vi "Main_13a.vi"() -> ()   [LabVIEW 2023]
panel:
  out "Array":cluster{"Array":bool[][]}[](array[cluster])
  out "Answer":i32
  in  "Puzzle":string=".####.#...##.#.\n...###.##.#.#..\n...###.##.#.#..\n.####.#...#..#.\n..##......#..#.\n#.#...#.##...##\n.#.#.#..##..##.\n#..##...#####.#\n.#.#.#.#..##.#.\n.....###.#.#..#\n.....###.#.#..#\n\n.#.###.....\n#..#.##...#\n.#.....#.#.\n.#.....#.#.\n#..#.##...#\n.#.###.....\n##.#..##.##\n#....##..#.\n.##.##.#.##\n...#..###.#\n...#..###.#\n.##.##.#.##\n#....##..#.\n####..##.##\n.#.###.....\n#..#.##...#\n.#.....#.#.\n\n###....##....\n####..#..#..#\n..###.####.##\n..#..######..\n...#.######.#\n#####.#.##.##\n##.#..#..#..#\n##....####...\n....#......#.\n.....#.##.#..\n##...##..##..\n...##.#..#.##\n##..###..###.\n\n.##.#...##.\n.#.########\n.##.#.#.##.\n#.##..#....\n####.##....\n####.##....\n#.##..#....\n.##.#.#.##.\n.#.########\n.##.#...##.\n..####.####\n.##.###.###\n.#..#.#.##.\n#.####..##.\n...#..#....\n\n.....##..#.\n.##..##.#.#\n#..#...####\n####.....##\n#..#.##....\n#####.....#\n#####.....#\n#..#.##....\n####.#...##\n#..#...####\n.##..##.#.#\n.....##..#.\n....##.##..\n\n#####..\n.##.#..\n.##....\n.##...#\n.##....\n#..####\n..#.#.#\n#####..\n#####.#\n.##...#\n.##.##.\n.##.##.\n.##...#\n\n.##.#.##.##.##.##\n.##.####....###..\n.##.#.#.#.##..##.\n#..#.#..#.#.##.#.\n....####...####..\n#..##.#...######.\n....#.#..........\n#..#.##.####..###\n#####...##......#\n....###..##.##.##\n####..###..####..\n.##..##..#.####.#\n#..##..##..#..#..\n.##..#.#.#..##..#\n####..####.####.#\n####.....###..###\n#..#..##.##.##.##\n\n.#..#.#.#####\n#.##.#.#.#.##\n#.##.#.#.#.##\n.#..#.#.#.###\n##..##..###..\n##.####.#####\n.##.#.#...###\n\n.###.#.###.###..#\n...####.####..#.#\n#..####.####..#.#\n.###.#.###.###..#\n...###..#..##....\n.#.#####.###..###\n#.#.#####.#.#####\n.##.###.#...###..\n.##.#.....##..##.\n#..##.####...##..\n#.#.#..#....#.###\n..#...#...##..##.\n##..#.######...##\n###.#.####..#..##\n...#..##..##...##\n###....##.#..#..#\n###....##.#..#..#\n\n##.###..####..#\n#.###.###.##..#\n..##...##..##.#\n..##...##..##.#\n#.###.###.##..#\n##.###..####..#\n....#####.#####\n##..#....#.#..#\n##.#..#.#...#..\n.##.#..##.#.###\n.##.#..##.#.###\n#..#..#.#...#..\n##..#....#.#..#\n\n.###.#....##....#\n#.##.##........##\n...###.#..##..#.#\n...###.#..##..#.#\n#.##.##........##\n.###.#....##....#\n.###..#.##..##.#.\n.###.#...####...#\n####.....####....\n###...##...#..##.\n.#..#.#.#.##.#.#.\n\n#.#..#.\n#.#..#.\n#......\n###..##\n##.##.#\n..####.\n#......\n##.....\n.##..##\n..#..#.\n..#..#.\n.##..##\n...##..\n\n##.#########..##.\n...#.####.#.##..#\n##.#...#..##..##.\n....#..###.##.#.#\n....#..###.##.#.#\n##.#...#..#...##.\n...#.####.#.##..#\n##.#########..##.\n##...####...##...\n###...##..###.#.#\n...#.#..##.#.....\n.........#####...\n....##..#.#.##.##\n...#.#.###.....#.\n...##..#.##.#.#.#\n##...##....#.####\n###....###......#\n\n..##.##.##......#\n.###....###....##\n#.###..###.####.#\n.##########.##.##\n...##..##........\n###......###..###\n.##########....##\n.#.######.#.##.#.\n.....##.....##...\n####.##.####..###\n...#....#........\n.##.#..#.##.....#\n..##.##.##......#\n\n####.##\n.##..#.\n..###.#\n.##.#.#\n###.#..\n##...##\n##...##\n#####..\n.##.#.#\n..###.#\n.##..#.\n####.##\n####.##\n.##..#.\n..###.#\n\n#.###..\n.....##\n..#....\n.#.##..\n..#.###\n..#..##\n.#.##..\n\n#..#.###....#####\n##.####.####.####\n#...###..#..#.##.\n..###.#.##.....#.\n..#....####..####\n...#.###.#.##.##.\n.#...###.#..#####\n.#.#...##.#......\n.##.##..#.....##.\n.#..#.#...##.#..#\n.#....##.##.##..#\n###..####.###....\n###..####.###....\n\n######.#.##....\n.####.#..##.##.\n.####.##..#....\n.####.#.#.#####\n#....#..####..#\n.####...#.#....\n..........##..#\n..##..#.#####.#\n######.#...####\n#.##.##.....##.\n.#..#...##.####\n..........#####\n#.##.#####.#..#\n\n#####.#\n##.##.#\n#.#.###\n...##.#\n######.\n......#\n......#\n######.\n...##.#\n#.#.###\n##.##.#\n\n.#..#.#####...#..\n#######.#.#.....#\n#....#...#.#...##\n######...###...##\n.#..#..###..#..##\n#....##..#...##.#\n.####..##.###.##.\n.#..#.##.###..#..\n#....#.#.##.##.#.\n.#..#.#...#.##...\n.####.##.#.#....#\n.......#.##.#.##.\n.......#.##.#.#..\n.####.##.#.#....#\n.#..#.#...#.##...\n\n##.####\n..#....\n###....\n.##....\n#.#....\n#.#....\n..#....\n###.##.\n#..####\n#.#####\n###....\n#..####\n.######\n##.####\n.#.....\n\n###.##....##.##\n##.##......##.#\n####...##...###\n....#.#..#.#...\n....#.....##...\n#####..##..####\n###..##..##..##\n###..#.##.#..##\n###..#....#..##\n#####.####.####\n..#.#..##..#.#.\n..#..#.##.#..#.\n##............#\n\n###.#.##.#.#.#.\n###.#.##.###.#.\n##..#...##....#\n.#..###.###..##\n#.#......###.##\n........##.##.#\n........##.##.#\n#.#......###.##\n.#..###.###..##\n##..#...##....#\n###.#.##.###.#.\n###.#.##.#.#.#.\n.#..#.#...#.###\n.....##.#.##.#.\n.#.###.#.###.##\n.#.#.....###.#.\n##....####.#.##\n\n###......###.\n##.######.###\n###.####.###.\n##..#..#..##.\n..##....##...\n###..##..###.\n####....#####\n####.##.####.\n##.##..##.##.\n#...####...#.\n...#....#....\n...#....#....\n..#.#..#.#..#\n\n.##..##.###..##\n.##.#...##.#.#.\n.##.#...##.#.#.\n.##..##.###..##\n#...#.#..####..\n.#.#....#.#....\n#..##..#..##...\n##....####..#..\n.#.....#.###..#\n..#....#.#...#.\n.##...#.#..#.##\n...##.#..######\n.###.......####\n.###.......####\n...##.#...#####\n\n.#........#.##.\n#.##.#...##.#.#\n###.####...##.#\n###.####..###.#\n#.##.#...##.#.#\n.#........#.##.\n...#.##.#.#.##.\n#.####.###.####\n.#...##.##.###.\n.....#..#.####.\n##.##.##..##..#\n.....#..#.....#\n##.##.#.#####..\n##.##.#.#####..\n.....#..#.....#\n##.##.##..##..#\n.....#..#.####.\n\n######.##.###\n.#..##.##.##.\n#.#.##.##.##.\n#.#..#.##.#..\n....#.####.#.\n#...#..##..#.\n####.#....#.#\n.###.######.#\n####.###.##.#\n....###..###.\n..###.####.##\n..###.####.##\n....###..###.\n\n..##..##..#\n..###.#....\n##....#....\n###.#.#.##.\n##.####.##.\n##...##.##.\n...##..####\n##.#####...\n...#.##....\n..#####.##.\n...#..##..#\n..#.#..####\n##.....####\n...##.#.##.\n..#####.##.\n.....#.#..#\n##.##...##.\n\n#......##.##.##\n..####..#####..\n..#..#...#..#..\n.######.##.#...\n..#..#....#####\n...##....######\n.........#.##..\n.##..##.#......\n####.####.#.###\n\n#......##......##\n..####....####...\n..#..#....#..#..#\n...##......##....\n################.\n.#....#..#....#..\n...##......##....\n.#....#..#....#..\n##....####....##.\n..#..#....#..#...\n..#..#....#..#..#\n##.##.####.##.##.\n###..######..###.\n..####....####...\n...##......##....\n####.######.#####\n.#.##.#..#.##.#.#\n\n...##.##.##..\n##..........#\n##..##..##..#\n..#.######.#.\n##...####...#\n...##.##.##..\n###..####..##\n##...####...#\n...##.#..##..\n....##..##...\n##..#.##.#..#\n\n.#.##.####.##.#..\n##..###..###..##.\n##..##....##..##.\n#.#.##....##.#.#.\n#.#.###..###.#.#.\n##...##..##...###\n#..#.##..##.#..##\n....#.#..#.#....#\n....#.#..#.#.....\n\n.##.#.....#...###\n###..#.####..####\n##....#..####....\n#..###..#.#..####\n..#.####.####.##.\n.##....##...#.##.\n.##....##...#.##.\n..#.####.####.##.\n#..###..#.#..####\n##....#..####....\n###..#.####..####\n\n##..#.#..#.#.\n##.###.##.###\n#######..####\n##..##....##.\n##.####..####\n#####..###.##\n####...##...#\n....###..###.\n..##..#..#..#\n..#..##..##..\n##.##.#..#.##\n###.###..###.\n...##.####.##\n##.###.##.###\n...#...##...#\n..#....##....\n.....#....#..\n\n..#.##.##\n..#..####\n#...#.##.\n#...#.##.\n..#..####\n..#.##.##\n######...\n#.##..#..\n.#.....#.\n###.###.#\n#.##..###\n.#..#..#.\n###.##...\n###..#...\n###..#...\n###..#...\n.#..#..#.\n\n###.###.##.\n###.###.##.\n##.#.##..#.\n....#.##.##\n.#.##.##.##\n###....####\n###.##..#..\n\n####.#..##..#.#\n.......######.#\n####.##.....#..\n####.##.....#..\n.......######.#\n####.#..##..#.#\n.##.####.#.#.#.\n######....#.#.#\n.......#....#..\n###...###.#####\n#..#..#####.###\n......##.##.#..\n.##.###.###...#\n####...###.####\n#####.###...#.#\n\n#####....\n#...#####\n#....####\n#..##..##\n#..##..##\n#....#.##\n#...#####\n#####....\n#..#..#..\n.#....###\n##.#..#..\n.#...####\n###.#.###\n##.#.....\n##...#.##\n\n....#.#.#......\n.....#.#####...\n....###..#.#...\n..#...#..##.###\n####...##..####\n.##...##.###.##\n#..#..#........\n#..###..##.....\n.....####...#..\n.##.#.#.###.###\n####.##.#.#.###\n.....#.#.....##\n########...####\n#..###..###..##\n.##.###.#..####\n\n.#.#..##.#.#.#.\n....##.....##..\n#.#.####..####.\n#..#..##.###...\n#..#..##.###...\n#.#.####.#####.\n....##.....##..\n.#.#..##.#.#.#.\n.#####..#..####\n#....#.#..##..#\n#..#.#..##.#..#\n#.##..#..#.#..#\n.####..##.#..#.\n.####..##.#..#.\n#.##..#..#.#..#\n#..#.#..##.#..#\n#....#.#..##..#\n\n#..#######..#.#..\n#.#...#.###..####\n##....###.###.###\n.........#.#.....\n.#.#..####...##..\n#.#.##.#.###...##\n#.#.#...####.....\n#.#.#...####.....\n#.#.##.#.###...##\n.#.#..####...#...\n.........#.#.....\n##....###.###.###\n#.#...#.###..####\n#..#######..#.#..\n##...#.####....##\n\n....######.\n###.....#.#\n###.....#.#\n.#..######.\n.#..######.\n###.....#.#\n###.....#.#\n....######.\n.#####.###.\n#..#......#\n##....##.##\n.#.#.#..#.#\n.####....##\n##...#.#.#.\n#...###..#.\n\n########..###\n....###....##\n....###.##.##\n####.........\n....####..###\n#..##..####..\n######.####.#\n#..#...#..#..\n####...####..\n.##.....##..#\n#..##########\n#..#..######.\n.##.#..#..#..\n\n#.##.####.#....\n#.##.####.#....\n##...##.##..###\n..#..#...#.#..#\n#.#....#.##...#\n.#.####.#...#.#\n####.#.#....###\n.##.#.####...##\n.##.#.####...##\n####.#.#.#..###\n.#.####.#...#.#\n#.#....#.##...#\n..#..#...#.#..#\n##...##.##..###\n#.##.####.#....\n\n###..##\n###..##\n#..##.#\n.##....\n.##....\n#..##.#\n####.##\n\n....#...#..#.\n.##..#..#.#.#\n####.##.##.#.\n###.###..#...\n#.#.#...###.#\n#.#.#...###.#\n###.###..#...\n####.##.##.#.\n.##..#..#.#.#\n....#...#.##.\n#.###.##.##.#\n#.###.##.##.#\n....#...#.##.\n.##..#..#.#.#\n####.##.##.#.\n\n..#..#........#\n...##....#.#...\n##....###...#.#\n##....##.###.#.\n...##...#.#.#..\n........#######\n##....##.#.....\n..............#\n#########.##.#.\n........#.#.##.\n#########..##..\n.######..##..#.\n..####..###..#.\n..####.....#...\n..####...##....\n\n..#####.###\n...####.###\n.....#.#...\n.####..##.#\n##...#..###\n##...#..###\n.####..##.#\n\n#..##.###.####.##\n########.##..##.#\n.##....##.####.##\n#######.#......#.\n####..##...#....#\n####..###########\n....#############\n......##.##..##.#\n#######..##..##..\n#..##.#...#..#...\n.##.#.##.##..##.#\n.##..###..#..#..#\n....#.##........#\n.....##.#.####.#.\n.##.#.##........#\n\n.##....#...#.#...\n.##....#...#.#...\n..#...###.#####..\n.####...#..#..##.\n##.###.#.....##..\n.....##.#..#.#.##\n.#.##....##.#.#..\n#..........####..\n#.....###.##...##\n\n#.###..##..\n.#..#.#..##\n###..##....\n###..##....\n.#..#.#.###\n#.###..##..\n####.#..###\n\n.....#.####..#..#\n.....#.####..#..#\n..#.#..###.#..#.#\n####..#####.##...\n..#.##..###.....#\n##...#.###.#..#.#\n###.#.#...#...###\n.###.....#.##..#.\n.###....##.##..#.\n\n...#...#..#.##..#\n#..##.#..####.##.\n.##..#.#..##..##.\n..##..###....#..#\n.#.....###.#.####\n###..#.#.##...##.\n###..#.####...##.\n\n##.##..\n..#....\n.#.#...\n##.####\n##.####\n...#...\n..#....\n##.##..\n#.#####\n##..#..\n.#.#...\n..#.#..\n###.###\n....###\n.##.#..\n#..#.##\n##...##\n\n###.#....#.##\n#..#.#..#.#..\n#..#.#..#.#..\n###.#....#.##\n#.###....###.\n.##...#....##\n...#.####.#..\n##..##..##..#\n..#..####..#.\n.##..####..##\n##..#....#..#\n..##.#..#.##.\n.##.#....#.##\n\n..#######\n...##.##.\n##.#.####\n#.#..#..#\n.#.##....\n#.##.#..#\n...######\n#..######\n#.##.#..#\n\n######.........\n.##..##..##..##\n.......##..##..\n.#.#...#.##..##\n#.#.##...#....#\n.##..#.....##..\n.##..#.....##..\n#.#.##...#....#\n.###...#.##..##\n\n####..#.##.#.\n###.#.#.##.#.\n#.##..#.##.#.\n....#..#..#..\n.#.###.####.#\n##..#.######.\n.#.##.#.##.#.\n#.##..######.\n#.##..######.\n.#.##.#.##.#.\n##..#.######.\n.#.###.####.#\n....#..#..#..\n#.##..#.##.#.\n#.#.#.#.##.#.\n####..#.##.#.\n.#..#.#.##.#.\n\n.#........#..\n#.###..###.##\n.#..####..#..\n#.#.#..#.#.##\n.#.#.##.#.#..\n.##..##..##..\n#...####...##\n..#.#..#.#...\n...#.##.#....\n#..#....#..#.\n..#.####.#...\n.##########..\n.#........#..\n#..#....#..##\n..##....##...\n\n.##..###...#...\n.##.##.########\n#.#.#..#..#..#.\n.#......###..##\n....######.##.#\n.#.##......##..\n##.#...###.##.#\n##.#...###.##.#\n.#.##......##..\n....######.##.#\n.#......###..##\n\n.##...##.\n#..#.###.\n####.....\n#..######\n.##..#..#\n.##.#####\n....#####\n\n.###...#####.###.\n..##...#..##..##.\n..##..#..#...#..#\n##..###.#.#.#.##.\n##..##.#.#......#\n##..###...##.###.\n........##.###..#\n.####.#....###..#\n#.##.###..#..###.\n.........#.#.#..#\n##..##.#.##..###.\n##..##.#.##..###.\n.........#.#.#..#\n\n....#......#...\n....###..###...\n.....######....\n##.#.#....#.#.#\n##.....##.....#\n..##..#..#..##.\n..####....###..\n\n.....#.#..#\n#####.#####\n#..########\n#..#.######\n#....#..##.\n.##.#..#..#\n#..#..#####\n\n#.##.#..#\n##..#.##.\n..###.##.\n..#...##.\n#.#...##.\n###......\n###......\n#.#...##.\n.##...##.\n\n.......#.\n.......#.\n.#..#.#..\n.####...#\n..##..#.#\n########.\n.####.#.#\n..##.....\n..##...#.\n#....#..#\n##..##.##\n######...\n.#..#.#.#\n#.##.###.\n#.##.##..\n....#...#\n######.##\n\n#..#..#........#.\n....##..#.##.#..#\n....##.#..##..#.#\n.....#...#..#...#\n####..#.##..##.#.\n.##.#####....####\n....#.#.##..##.#.\n...######....####\n######..##..##..#\n\n###.#..\n####..#\n..#....\n###.##.\n...#..#\n..#.##.\n###.##.\n###....\n..#.##.\n\n.#..###....#...\n##...#...###...\n.#..#..##...#.#\n.#..#..##...#.#\n##...#....##...\n.#..###....#...\n###..###..#.#.#\n#.##.#.#.#####.\n#......##...#.#\n###....#.#.#.#.\n###....#.#.#.#.\n#......##...#.#\n#.##.#.#.#####.\n###..###..#.#.#\n.#..###....#...\n##...#....##...\n.#..#..##...#.#\n\n..##.#.\n##.##..\n..##.#.\n...##.#\n#.#####\n..###.#\n..#.##.\n###.###\n##...#.\n..####.\n..####.\n##...#.\n###.###\n\n.##.#...#.##.\n#.####.####.#\n####...#.#..#\n.##.#.######.\n######...##.#\n.....#..#.#..\n.....#..#.#..\n######...##.#\n.##.#.######.\n\n.###.#.#.\n...#.##..\n##.....##\n###..#.#.\n#.#..##..\n...#..##.\n.......#.\n.......#.\n...##.##.\n...##.##.\n.......#.\n.......#.\n...#..##.\n\n...##....####.##.\n.##..###.#...####\n###..###.####.##.\n.######.#....####\n########....#.##.\n..#..#..##..#....\n.##..##...#......\n..#..#..##.###..#\n#.####.##.#......\n\n#.#..#####..#..\n##.##.####..###\n#......#.##.#.#\n###..####.##...\n#.#..#.###...#.\n.#.##.#.#.#.###\n##.##.##..#.###\n.##..##.#####..\n#......#.##....\n#......#.##....\n.##..##.#####..\n##.##.##..#.###\n.#.##.#.#.#.###\n#.#..#.###...#.\n###..####.##...\n#......#.##.#.#\n##.##.####..###\n\n####..#####\n.....#..###\n#..####.#..\n.......##..\n#..#..#.###\n####.......\n.....#.#.##\n#..##..#...\n.##...##..#\n.......###.\n.##..##..##\n....#....##\n####.#.##.#\n#####.####.\n#####.###..\n\n#..#.####.#.#..\n#.#####.#.#####\n##.#...##.#...#\n#..#.##...#.##.\n#..#.##...#.##.\n##.#...##.#...#\n#.#####.#.#####\n#..#.####.#.#..\n#..#.######.###\n.....####....##\n.##.....##.####\n......#.##..##.\n......#.##..##.\n.##.....##.####\n.....####.....#\n#..#.######.###\n#..#.####.#.#..\n\n#.#...###\n#.#####..\n.###.....\n.###.....\n#.#####..\n#.#...###\n.#.....#.\n.#..###.#\n.#..###.#\n.#.....#.\n#.#...###\n#.#####..\n.#.#.....\n\n..........###\n..##....#.###\n..##....#..##\n..........###\n.####...#....\n.####.######.\n##..##.######\n.####.....##.\n.####.##.###.\n\n######..##.\n.#..#..#..#\n#######.##.\n######..##.\n.####.##..#\n.####.#....\n.####...##.\n.#..#.#####\n##..#######\n.####.#....\n#.##.##....\n..##....##.\n.#..#.#####\n##..##..##.\n.####...##.\n#.##.##..#.\n#....###..#\n\n#...#..#....#.##.\n..........###.##.\n....#.#.###..#..#\n.###...######.##.\n.###....#####.##.\n....#.#.###..#..#\n..........###.##.\n#...#..#....#.##.\n##.###.###...####\n#......#...#.#..#\n..#..##..........\n.###.###.##...##.\n..##.#####..#####\n....#.##.#.##....\n....##.#..#.##..#\n...#####....##..#\n....#.###..#.####\n\n...######...#\n##.##..##.##.\n##.#....#.###\n####.##.#####\n#..........##\n....#........\n.####..####.#\n.#.##..##.#..\n#....##....##\n#..........##\n....####.....\n##.##..##.###\n##.##..##.###\n\n###..##\n##.#.#.\n..#...#\n##..#..\n#####.#\n###..#.\n###....\n\n#####.#\n...####\n.##....\n...#..#\n#.#....\n.######\n###....\n###....\n.######\n\n..#..####..\n####.####.#\n####.####.#\n..#...###..\n##...#.#.#.\n...####...#\n....#...##.\n..#.###.#.#\n#######.##.\n...#...##.#\n..#.#.#...#\n####.#....#\n.....#..#.#\n\n######..#\n..##...#.\n##..##.#.\n#....###.\n#....##..\n##..##.#.\n..##...#.\n\n#.##..#\n#####..\n##.##..\n##.##..\n#####..\n#.##..#\n.###.##\n.#.##..\n.###.##\n.##..##\n#.#.###\n.#.....\n##.##..\n.######\n.#.####\n\n####..#..#..###\n..#.########.#.\n####...##...###\n...##########..\n..#..........#.\n###.########.##\n..#..##..##..#.\n##..#.####.#..#\n##.#.##..##.#.#\n###.###..###.##\n####.##..##.###\n..#....###...#.\n..##.#....#.##.\n##..##.##.##..#\n...##########..\n######.##.#####\n###..........##\n\n#.....#...#..#...\n##.#...#..#..#..#\n##.###.##########\n##.##.###########\n#.##...#.#.##.#.#\n#.#..............\n..##.....##..##..\n##..#......##....\n##.##.#.#.####.#.\n##..#.#.#.####.#.\n##..#......##....\n\n......#.##.#...\n#.##.#......#.#\n......####.#...\n.#..#.#....#.#.\n##..###.##.###.\n.#..#.#....#.#.\n#....##....##..\n.####..####..##\n.####.#....#.##\n\n#####.#.##.#.\n...##...##.#.\n...##...##.#.\n#####.####.#.\n####...#....#\n####.....###.\n##....###.##.\n##...##...###\n..###...##.#.\n.....#.#.##..\n...#.##......\n####..#####..\n###.#....##..\n..######..###\n....##...#..#\n\n.##.###....####\n#......#..#####\n..#..#..#.##..#\n#...##.####....\n.###...####....\n.###...####....\n#...##.####....\n..#..#..#.##..#\n#.....##..#####\n\n#..##..#.#.#..#\n....#.#.##.##.#\n....#.#.#.####.\n####.#.....##.#\n.##...#.#..###.\n.##...#.#..###.\n####.#.....##.#\n....#.#.#.####.\n....#.#.#..##.#\n#..##..#.#.#..#\n####.#...##.#.#\n#####..#.###..#\n.....#.#.#.##..\n#..##.##.###.#.\n#..#...##.#.#.#\n....##.###.#..#\n.##.###.....##.\n\n.#..#.##.####..##\n#..##..#.#.#...##\n#...#.#.##.#.##.#\n##..###....#.###.\n.###...#.#.####.#\n.###...#.#.####.#\n##..##.....#.###.\n#...#.#.##.#.##.#\n#..##..#.#.#...##\n.#..#.##.####..##\n.#....###..##...#\n#.#.######..#####\n...#.#..##...####\n.#.#####.....##..\n##.#.#.##.###....\n##.#.#.##.###....\n.#.#####.....##..\n\n.#..#.#.#.##.\n##..##.#.....\n#....#.#.####\n#.##.#.#..##.\n..##..#......\n##..##.##.##.\n#....#.#..##.\n######..#####\n..##....##..#\n#.##.#..##..#\n.........####\n..##..#.##..#\n.#..#..##....\n....#...#####\n##..##..#.##.\n.####.####..#\n##..##.######\n\n#....#..#\n###..#...\n##.######\n..##..#.#\n..####.##\n##...####\n##.#..###\n.....#.#.\n..##...#.\n...#.###.\n####..###\n......###\n...#....#\n#####.#.#\n..#.#..#.\n..#.#..#.\n#####.#.#\n\n#######...#....#.\n###.#..##..#..#..\n#.###.#..#..##..#\n#.###.#..#..##..#\n###.#..##..#..#..\n#######...#....#.\n#...#.#.##.####.#\n..#.#.#.##.#..###\n#.#...#.###....##\n.######.....##...\n#..#.#.##.##..##.\n.##..#.##.#....#.\n#.##..######..###\n#...#.#..########\n#.###.#..........\n\n#..#..#..##..#..#\n#.###############\n####..##....##..#\n##.####......####\n..#####..##..####\n#.##..#..##..#..#\n###.####.##.####.\n##.#..#......#..#\n.###..#.#..#.#..#\n.#.#..#..##..#..#\n##.####......####\n.##.##.#.##.#.##.\n.######.####.####\n\n#.#....#.\n###..#..#\n###..#..#\n#.#....#.\n.####..#.\n..##..###\n..#.#..#.\n#..#..##.\n.###.###.\n...#..#..\n...#....#\n###.#.###\n....#.#.#\n##.#.##.#\n##.####.#\n#..####.#\n##.#.##.#\n\n......#\n#####.#\n......#\n####.#.\n.##...#\n#..#.#.\n.###.##\n.....#.\n.##....\n.##....\n.....#.\n\n...###.#.....##..\n#.######.#.......\n#.##.###.#.......\n...###.#.....##..\n.#..##..#.###..##\n#..###.####...###\n#####.#...#.##...\n#####.#..###.####\n#########.#.#####\n.#####....##..###\n##.#..#..####..##"
  in  "Example":string="#.##..##.\n..#.##.#.\n##......#\n##......#\n..#.##.#.\n..##..##.\n#.#.##.#.\n\n#...##..#\n#....#..#\n..##..###\n#####.##.\n#####.##.\n..##..###\n#....#..#"
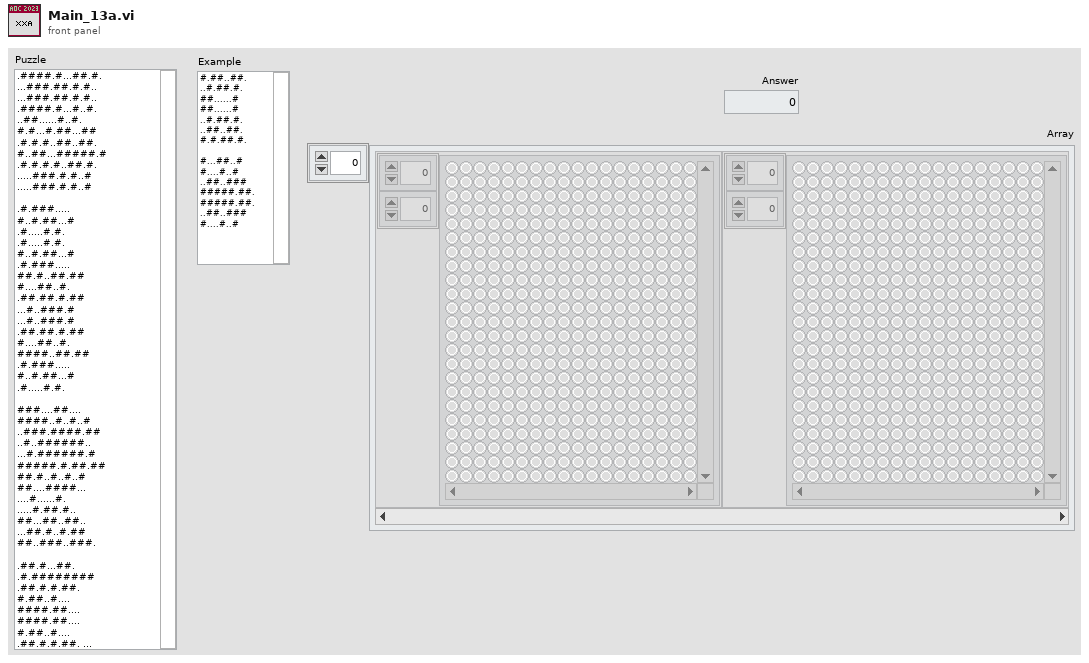
[diagram p1: front panel]
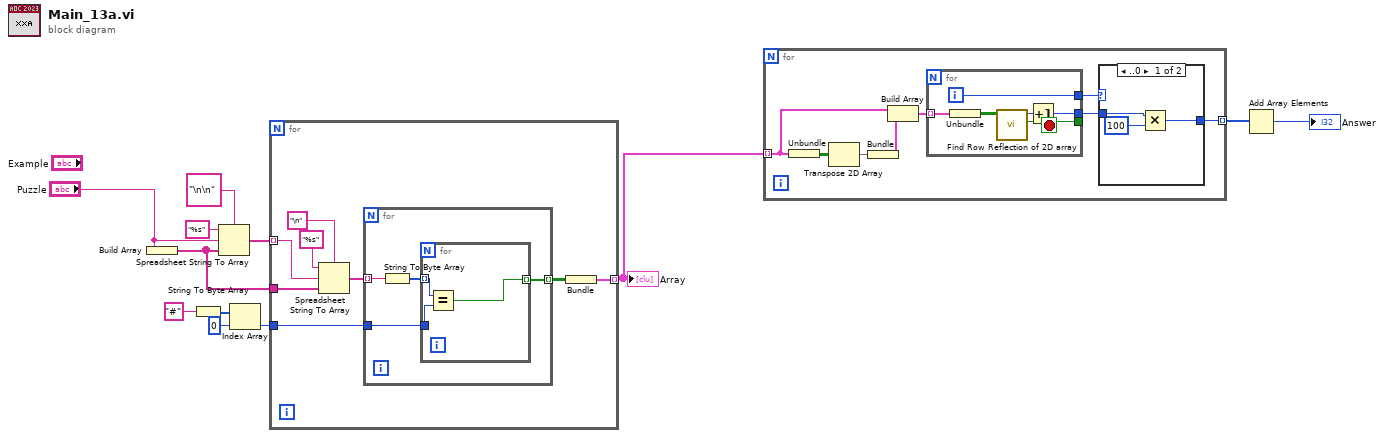
[diagram p0: block diagram]
diagram:
  n1 = Build Array("Puzzle") -> (w9:string[])
  n2 = String To Byte Array(string="#" ("format string")) -> (unsigned byte array=w7:u8[])
  n3 = Spreadsheet String To Array(delimiter (Tab)="\n\n", format string="%s", spreadsheet string="Puzzle", array type (2D Dbl)=w9) -> (array=w10:string[])
  n4 = Index Array(array=w7, index=0) -> (element=w5:u8)
  n5 = for {
    tunnel: w10 -> [w19] mode=indexing
    tunnel: w9 -> [w17]
    tunnel: [w15] -> w4 mode=indexing
    tunnel: w5 -> [w14]
    n6 = Spreadsheet String To Array(delimiter (Tab)="\n", format string="%s", spreadsheet string=w19, array type (2D Dbl)=w17) -> (array=w16:string[])
    n7 = for {
      tunnel: w16 -> [w24] mode=indexing
      tunnel: w14 -> [w22]
      tunnel: [w21] -> w13 mode=indexing
      n8 = String To Byte Array(string=w24) -> (unsigned byte array=w23:u8[])
      n9 = for {
        tunnel: w23 -> [w26] mode=indexing
        tunnel: w22 -> [w27]
        tunnel: [w25] -> w21 mode=indexing
        n10 = Equal?(x=w26, y=w27) -> (x = y?=w25:bool)
      }
    }
    n11 = Bundle(w13) -> (w15:cluster{bool[][]})  [unwired: 1 in]
  }
  "Array" <- w4
  n12 = for {
    tunnel: w4 -> [w33] mode=indexing
    tunnel: [w28] -> w3 mode=indexing
    n13 = Unbundle(w33) -> (w35:bool[][])
    n14 = Transpose 2D Array(2D array=w35) -> (transposed array=w34:bool[][])
    n15 = Bundle(w34) -> (w32:cluster{bool[][]})  [unwired: 1 in]
    n16 = Build Array(w33, w32) -> (w31:cluster{bool[][]}[])
    n17 = for {
      tunnel: [w42] -> _
      tunnel: [w40] -> w29
      tunnel: w31 -> [w44] mode=indexing
      tunnel: [w43] -> w30
      i -> [w43]
      stop <- w42 stop-if-true
      n18 = Unbundle(w44) -> (w41:bool[][])
      n19 = call "Find Row Reflection of 2D array.vi"("2D array"=w41) -> ("Reflection found"=w42:bool, "Row index of reflection"=w45:i32)  [unwired: 9 in]
      n20 = Increment(x=w45) -> (x+1=w40:i32)
    }
    n21 = case shown="..0" w30 {
      tunnel: w29 -> [w38 w39]
      tunnel: [w36 w39] -> w28
      frame ..0 {
        n22 = Multiply(x=w38, y=100) -> (x*y=w36:i32)
      }
      frame 1.. {
      }
    }
  }
  n23 = Add Array Elements(numeric array=w3) -> (sum=→"Answer":i32)
